vi "observacao_queued.vi"() -> ()   [LabVIEW 2012, in "Shared_160.lvlib"] (continued)
                w579 = u16 7 items=["Alarme", "Atencao", "Erro", "Ocupado", "TBD", "LCB", "Trapeira", "Paravento", "DomoRap", "DomoCW", "DomoCCW", "TBD", "Em movimento", "TBD"] ("NomeStatus")
                # "Aqui também caberia um Timeout?"
                # "Também poderia ser testado o bit \"Em movimento\".\nNeste caso o código do \"IF\" deve ser permutado."
                # "Aguarda abaixamento Paravento"
                n668 = call "Bit Status CUP.vi"("NomeStatus"=w579) -> ("StatBit"=w581:bool)
                n669 = case shown="True" w581 {
                  tunnel: [5 6] -> w580
                  frame False {
                    # "Ainda movendo...\nAGUARDAR"
                  }
                  frame True {
                    # "Paravento abaixado."
                  }
                }
              }
              frame 6 {
                w584 = u16 6 items=["Alarme", "Atencao", "Erro", "Ocupado", "TBD", "LCB", "Trapeira", "Paravento", "DomoRap", "DomoCW", "DomoCCW", "TBD", "Em movimento", "TBD"] ("NomeStatus")
                # "Verifica Trapeira"
                n670 = call "Bit Status CUP.vi"("NomeStatus"=w584) -> ("StatBit"=w585:bool)
                n671 = Not(x=w585) -> (.not. x?=w589:bool)
                n672 = And(x=w589, y="ChkOpenShutter") -> (x .and. y?=w587:bool)
                n673 = case shown="True" w587 {
                  tunnel: [0 w594] -> w590
                  tunnel: w586 -> [_ w595]
                  frame False {
                    # "Verificar Paravento"
                    # "Trapeira aberta\nou desabilitada"
                    n674 = call "TickTimeout.vi"() -> ("msTick"=w591:u32)  [unwired: 2 in, 2 out]
                    n675 = local write "TimeoutCUP"(w591) -> ()
                    n676 = global write "Global_Telescopio.vi" "T cup"(w591) -> ()
                    "Dome on Target" <- TRUE
                  }
                  frame True {
                    # "Abrir Trapeira"
                    n677 = case shown="False" w595 {
                      tunnel: [7 w600] -> w594
                      frame False {
                        w599 = u16 4 items=["ZERO", "AH", "DEC", "TUBO", "CUP"] ("Controlador")
                        # "Aguardar abertura Trap."
                        # "CLP Pronto"
                        n678 = call "Monta Comando.vi"("Comando"="ABRIR", "Dispositivo"="TRAPEIRA" ("Comando"), "Controlador"=w599) -> ()  [unwired: 4 in, 3 out]
                      }
                      frame True {
                        # "CLP Busy"
                        n679 = local read "TimeoutCUP"() -> (w602:u32)
                        n680 = call "TickTimeout.vi"("msInicial"=w602, "msTimeout"=u32 5000) -> ("Timeout"=w601:bool)  [unwired: 2 out]
                        n681 = case shown="True" w601 {
                          tunnel: [6 3] -> w600
                          frame False {
                          }
                          frame True {
                          }
                        }
                      }
                    }
                  }
                }
              }
              frame 7 {
                w606 = u16 6 items=["Alarme", "Atencao", "Erro", "Ocupado", "TBD", "LCB", "Trapeira", "Paravento", "DomoRap", "DomoCW", "DomoCCW", "TBD", "Em movimento", "TBD"] ("NomeStatus")
                # "Aqui também caberia um Timeout?"
                # "Aguarda abertura Trapeira"
                # "Também poderia ser testado o bit \"Em movimento\".\nNeste caso o código do \"IF\" deve ser permutado."
                n682 = call "Bit Status CUP.vi"("NomeStatus"=w606) -> ("StatBit"=w607:bool)
                n683 = case shown="True" w607 {
                  tunnel: [7 0] -> w608
                  frame False {
                    # "Ainda movendo...\nAGUARDAR"
                  }
                  frame True {
                    w611 = TRUE ("Dome on Target")
                    # "Trapeira aberta.\nFIM"
                    n684 = call "TickTimeout.vi"() -> ("msTick"=w610:u32)  [unwired: 2 in, 2 out]
                    n685 = local write "Dome on Target"(w611) -> ()
                    n686 = local write "RefreshShutterState"(w611) -> ()
                    n687 = local write "TimeoutCUP"(w610) -> ()
                    n688 = global write "Global_Telescopio.vi" "T cup"(w610) -> ()
                  }
                }
              }
            }
            n689 = case shown="True" w470 {
              tunnel: w459 -> [w490 _]
              tunnel: [w489 "POINT" ("Boolean Text.Text")] -> w458
              frame False {
                n690 = case shown="True" w490 {
                  tunnel: ["POINT" ("Boolean Text.Text") "STOP" ("Boolean Text.Text")] -> w489
                  frame False {
                  }
                  frame True {
                  }
                }
              }
              frame True {
                w493 = TRUE
                # "MUDANÇA:\n22/6/2011 \nHab. Guider"
                n691 = local read "ChkDomeEnable"() -> (w494:bool)
                n692 = global write "Global_Telescopio.vi" "Botão GO = STOP"(FALSE) -> ()
                n693 = local write "LED GUIDER"(w493) -> ()
                n694 = local write "GUIDER"(w493) -> ()
                n695 = local write "DOME"(w494) -> ()
              }
            }
            n696 = Tick Count (ms)() -> (millisecond timer value=w451:u32)
            n697 = Subtract(x=w451, y=w457) -> (x-y=w450:u32)
            n698 = Less?(x=w450, y=w452) -> (x < y?=w453:bool)
            n699 = control-ref of="BtTargetPoint"() -> (w487:refnum<vi>)
            n700 = case shown="True" w453 {
              tunnel: w452 -> [_ w488]
              frame False {
              }
              frame True {
                n701 = Wait Until Next ms Multiple(millisecond multiple=w488) -> ()  [unwired: 1 out]
              }
            }
            n702 = property class="Bool"(reference=w487, "Boolean Text.Text"=w458) -> ()  [unwired: 1 in, 2 out]
            n703 = call "PROTECAO.vi"("Estado In"=w463) -> ("Estado Out"=w462:i32)  [unwired: 2 in]
            n704 = local write "statCUP"(w462) -> ()
            "statCUP 2" <- "statCUP"
            "Erro Lim" <- 15 ("y")
            "Erro PROTEC" <- 10 ("y")
          }
          frame #4 {
            # "CHECA FINAL DO APONTAMENTO"
            # "ascensão reta = tempo sideral - ângulo horário (2)"
            n705 = local read "LedPointing"() -> (w909:bool)
            n706 = case shown="True" w909 {
              frame False {
                n707 = property on="DOME" class="Bool (strict)"("Disabled"=u8 0) -> ()  [unwired: 2 in, 2 out]
              }
              frame True {
                n708 = local read "statCUP"() -> (w914:i32)
                n709 = local read "statAH"() -> (w913:i32)
                n710 = local read "statDEC"() -> (w915:i32)
                n711 = Compound Arithmetic op=ADD(w914, w913, w915) -> (w916:i32)
                n712 = Greater Than 0?(x=w916) -> (x > 0?=w912:bool)
                n713 = case shown="False" w912 {
                  selector: w912 -> [w917 _]
                  frame False {
                    w920 = TRUE
                    n714 = local read "ChkPointPrecessed"() -> (w918:bool)
                    n715 = local read "StrPointObjName"() -> (w923:string)
                    n716 = local read "StrPointObjRA"() -> (w922:string)
                    n717 = local read "StrPointObjDEC"() -> (w921:string)
                    n718 = local write "LedPointing"(w917) -> ()
                    n719 = property on="LedPointing" class="Bool (strict)"("Visible"=w917) -> ()  [unwired: 2 in, 2 out]
                    n720 = case shown="True" w918 {
                      tunnel: ["2000.0" ("Saída") w925] -> w919
                      frame False {
                      }
                      frame True {
                        n721 = call "Calcula epoch.vi"() -> ("epoch"=w928:dbl)  [unwired: 2 in]
                        n722 = Number To Fractional String(number=w928, precision (6)=i16 1) -> (F-format string=w926:string)  [unwired: 2 in]
                        n723 = call "Comma_to_Point.vi"("Lat_A"=w926) -> ("Saída"=w925:string)
                      }
                    }
                    n724 = global write "Global_Telescopio.vi" "NAME OBJETO"(w923) -> ()
                    n725 = global write "Global_Telescopio.vi" "DEC AQUIS"(w921) -> ()
                    n726 = global write "Global_Telescopio.vi" "RA AQUIS"(w922) -> ()
                    n727 = local write "Processa Centragem"(w920) -> ()
                    n728 = property on="LedPointWorkArea" class="Bool (strict)"("Visible"=w920) -> ()  [unwired: 2 in, 2 out]
                    n729 = global write "Global_Telescopio.vi" "EPOCH AQUIS"(w919) -> ()
                  }
                  frame True {
                  }
                }
              }
            }
            n730 = local read "VARIABLE \nTRACKING"() -> (w910:bool)
            n731 = case shown="False" w910 {
              frame False {
              }
              frame True {
                n732 = local write "DEC"("DECTARGET") -> ()
                n733 = local write "RA"("AHTARGET") -> ()
              }
            }
          }
          frame #5 {
            # "PROCESSO OBJETO CENTRADO"
            n734 = case shown="True" "Processa Centragem" {
              frame False {
              }
              frame True {
                w937 = u16 3 items=["Alarme", "Atencao", "Erro", "Ocupado", "Protecao", "Embreagem", "Tracking", "Var. Track", "Rápido", "Ligeiro", "Médio", "Lento", "Em movimento", ""] ("NomeStatus")
                w938 = u16 3 items=["Alarme", "Atencao", "Erro", "Ocupado", "Protecao", "Embreagem", "Tracking", "Var. Track", "Rápido", "Ligeiro", "Médio", "Lento", "Em movimento", ""] ("NomeStatus")
                # "Roda case interno quando \nos controladores AH e DEC\nestiverem desocupados."
                n735 = call "Bit Status AH.vi"("NomeStatus"=w938) -> ("StatBit"=w936:bool)
                n736 = call "Bit Status DEC.vi"("NomeStatus"=w937) -> ("StatBit"=w935:bool)
                n737 = Or(x=w936, y=w935) -> (x .or. y?=w932:bool)
                n738 = case shown="False" w932 {
                  selector: w932 -> [w957 _]
                  tunnel: "INDEXER" ("Comando") -> [w959 _]
                  tunnel: "ZERAR" ("Comando") -> [w958 _]
                  frame False {
                    w945 = u16 1 items=["ZERO", "AH", "DEC", "TUBO", "CUP"] ("Controlador")
                    w946 = u16 2 items=["ZERO", "AH", "DEC", "TUBO", "CUP"] ("Controlador")
                    w939 = 0.0 ("AcumAG DEC")
                    # "PROCESSOPRECESSÃO"
                    # "PROCESSO ZERA POS_MOTOR"
                    # "Precessão"
                    n739 = local read "PM_RA"() -> (w951:string)
                    n740 = local read "Temp amb"() -> (w954:string)
                    n741 = local read "hum local"() -> (w952:string)
                    n742 = local read "MeanDEC"() -> (w955:string)
                    n743 = local read "pressão atm"() -> (w953:string)
                    n744 = local read "MeanRA"() -> (w956:string)
                    n745 = local read "PM_DEC"() -> (w950:string)
                    n746 = call "Monta Comando.vi"("Comando"=w958, "Dispositivo"=w959, "Controlador"=w945) -> ()  [unwired: 4 in, 3 out]
                    n747 = call "Monta Comando.vi"("Comando"=w958, "Dispositivo"=w959, "Controlador"=w946) -> ()  [unwired: 4 in, 3 out]
                    n748 = call "PrecessFortran.vi"("Asc reta"=w956, "Var RA"=w951, "Declinação"=w955, "Temperatura (Kelvin)"=w954, "Pressao atmosferica (mB)"=w953, "Humidade relativa (0 a 1)"=w952, "Var DEC"=w950) -> ("Observed RA (radians)"=w949:dbl, "Observed Dec (radians)"=w948:dbl)  [unwired: 2 in, 5 out]
                    n749 = local write "Processa Centragem"(w957) -> ()
                    n750 = global write "Global_Telescopio.vi" "LatchPrecRA"(w949) -> ()
                    n751 = global write "Global_Telescopio.vi" "LatchPrecDEC"(w948) -> ()
                    n752 = global read "Global_Telescopio.vi" "Sideral Time"() -> (w942:dbl)
                    n753 = global read "Global_Telescopio.vi" "PosDEC"() -> (w944:dbl)
                    n754 = global read "Global_Telescopio.vi" "PosAH"() -> (w943:dbl)
                    n755 = Subtract(x=w942, y=w943) -> (x-y=w941:dbl)
                    n756 = local write "LatchDeslocDEC"(w944) -> ()
                    n757 = local write "LatchDeslocRA"(w941) -> ()
                    n758 = global write "Global_Telescopio.vi" "AcumPrecDEC"(w939) -> ()
                    n759 = global write "Global_Telescopio.vi" "LatchAG RA"(w939) -> ()
                    n760 = global write "Global_Telescopio.vi" "AcumAG DEC"(w939) -> ()
                    n761 = global write "Global_Telescopio.vi" "AcumPrecRA"(w939) -> ()
                    n762 = global write "Global_Telescopio.vi" "LatchAG DEC"(w939) -> ()
                    n763 = global write "Global_Telescopio.vi" "AcumAG RA"(w939) -> ()
                    n764 = global write "Global_Telescopio.vi" "ObjCentrado"(TRUE) -> ()
                    n765 = property on="Calagem" class="Bool"("Disabled"=u8 0) -> ()  [unwired: 2 in, 2 out]
                  }
                  frame True {
                  }
                }
              }
            }
          }
          frame #6 {
            w963 = u16 2 items=["Alarme", "Atencao", "Erro", "Ocupado", "TBD", "LCB", "Trapeira", "Paravento", "DomoRap", "DomoCW", "DomoCCW", "TBD", "Em movimento", "TBD"] ("NomeStatus")
            w964 = u16 3 items=["Alarme", "Atencao", "Erro", "Ocupado", "TBD", "LCB", "Trapeira", "Paravento", "DomoRap", "DomoCW", "DomoCCW", "TBD", "Em movimento", "TBD"] ("NomeStatus")
            w968 = u16 3 items=["Alarme", "Atencao", "Erro", "Ocupado", "Protecao", "Embreagem", "Tracking", "Var. Track", "Rápido", "Ligeiro", "Médio", "Lento", "Em movimento", ""] ("NomeStatus")
            w969 = u16 3 items=["Alarme", "Atencao", "Erro", "Ocupado", "Protecao", "Embreagem", "Tracking", "Var. Track", "Rápido", "Ligeiro", "Médio", "Lento", "Em movimento", ""] ("NomeStatus")
            w977 = "ERROS" ("Comando")
            w980 = u16 2 items=["Alarme", "Atencao", "Erro", "Ocupado", "Protecao", "Embreagem", "Tracking", "Var. Track", "Rápido", "Ligeiro", "Médio", "Lento", "Em movimento", ""] ("NomeStatus")
            w981 = u16 2 items=["Alarme", "Atencao", "Erro", "Ocupado", "Protecao", "Embreagem", "Tracking", "Var. Track", "Rápido", "Ligeiro", "Médio", "Lento", "Em movimento", ""] ("NomeStatus")
            w978 = "PROG" ("Comando")
            # "LOGTCS ERROS"
            n766 = call "Bit Status AH.vi"("NomeStatus"=w981) -> ("StatBit"=w971:bool)
            n767 = call "Bit Status AH.vi"("NomeStatus"=w969) -> ("StatBit"=w967:bool)
            n768 = call "Bit Status DEC.vi"("NomeStatus"=w980) -> ("StatBit"=w970:bool)
            n769 = call "Bit Status DEC.vi"("NomeStatus"=w968) -> ("StatBit"=w966:bool)
            n770 = call "Bit Status CUP.vi"("NomeStatus"=w963) -> ("StatBit"=w979:bool)
            n771 = call "Bit Status CUP.vi"("NomeStatus"=w964) -> ("StatBit"=w976:bool)
            n772 = Not(x=w976) -> (.not. x?=w975:bool)
            n773 = Not(x=w967) -> (.not. x?=w973:bool)
            n774 = Not(x=w966) -> (.not. x?=w974:bool)
            n775 = And(x=w979, y=w975) -> (x .and. y?=w962:bool)
            n776 = And(x=w971, y=w973) -> (x .and. y?=w972:bool)
            n777 = And(x=w970, y=w974) -> (x .and. y?=w965:bool)
            n778 = And(x=FALSE, y=w962) -> (x .and. y?=w961:bool)
            n779 = case shown="True" w965 {
              selector: w965 -> [_ w990]
              tunnel: w978 -> [_ w991]
              tunnel: w977 -> [_ w987]
              frame False {
              }
              frame True {
                w988 = u16 2 items=["ZERO", "AH", "DEC", "TUBO", "CUP"] ("Controlador")
                n780 = call "Monta Comando.vi"("Comando"=w987, "Dispositivo"=w991, "Controlador"=w988) -> ("Resposta"=w989:string)  [unwired: 4 in, 2 out]
                n781 = call "Envia LOG.vi"("Error message"=w989, "Controlador"=w988, "Log de erro"=w990) -> ()  [unwired: 5 in, 2 out]
              }
            }
            n782 = case shown="True" w961 {
              selector: w961 -> [_ w985]
              tunnel: w978 -> [_ w986]
              tunnel: w977 -> [_ w982]
              frame False {
              }
              frame True {
                w983 = u16 4 items=["ZERO", "AH", "DEC", "TUBO", "CUP"] ("Controlador")
                n783 = call "Monta Comando.vi"("Comando"=w982, "Dispositivo"=w986, "Controlador"=w983) -> ("Resposta"=w984:string)  [unwired: 4 in, 2 out]
                n784 = call "Envia LOG.vi"("Error message"=w984, "Controlador"=w983, "Log de erro"=w985) -> ()  [unwired: 5 in, 2 out]
              }
            }
            n785 = case shown="True" w972 {
              selector: w972 -> [_ w995]
              tunnel: w978 -> [_ w996]
              tunnel: w977 -> [_ w992]
              frame False {
              }
              frame True {
                w993 = u16 1 items=["ZERO", "AH", "DEC", "TUBO", "CUP"] ("Controlador")
                n786 = call "Monta Comando.vi"("Comando"=w992, "Dispositivo"=w996, "Controlador"=w993) -> ("Resposta"=w994:string)  [unwired: 4 in, 2 out]
                n787 = call "Envia LOG.vi"("Error message"=w994, "Controlador"=w993, "Log de erro"=w995) -> ()  [unwired: 5 in, 2 out]
              }
            }
          }
          frame #7 {
            # "MASSA DE AR"
            # "z'"
            # "z * (1 - 0,0012* (z* z -1) )"
            # "(z* z -1)"
            # "z"
            # "O Hour Angle é calculado com essa equação (AH = TS - RA), \nsendo TS o tempo sideral que você fica calculando o tempo todo e RA a \ncoordenada que vem do quadro TARGET da aba POINTING."
            # "Coslat"
            # "Sinlat"
            # "MASSA DE AR\n# define LAT -22,534444444444 / / Lat itude do telescópio\n# define SINLAT -0,383238771 / / Seno da Lat itude\n# define COSLAT 0,923649308 / / Cosseno da Lat itude\ndouble airmass (double ah, double delta) / / ângulos dos eixos AH e DEC em radianos\n{ double z;\nz = 1./ (SINLAT* sin(delta) + COSLAT* cos(delta) * cos(ah) ) ;\nz = z * (1 - 0,0012* (z* z -1) ) ;\nif (z > = 10) z = 9.999;\nif (z < 0) z = 0;\nreturn (z) ;\n}"
            n788 = global read "Global_Telescopio.vi" "AH_now"() -> (w997:dbl)
            n789 = global read "Global_Telescopio.vi" "delta_now"() -> (w998:dbl)
            n790 = Cosine(x=w998) -> (cos(x)=w1018:dbl)
            n791 = Sine(x=w998) -> (sin(x)=w1020:dbl)
            n792 = Cosine(x=w997) -> (cos(x)=w1016:dbl)
            n793 = Multiply(x=0.923649308 ("Delta=DEC"), y=w1018) -> (x*y=w1017:dbl)
            n794 = Multiply(x=-0.383238771 ("Delta=DEC"), y=w1020) -> (x*y=w1015:dbl)
            n795 = Multiply(x=w1017, y=w1016) -> (x*y=w1014:dbl)
            n796 = Add(x=w1015, y=w1014) -> (x+y=w1013:dbl)
            n797 = Reciprocal(x=w1013) -> (1/x=w1005:dbl)
            n798 = Subtract(x=w1005, y=1.0) -> (x-y=w1011:dbl)
            n799 = Multiply(x=w1005, y=w1011) -> (x*y=w1010:dbl)
            n800 = Multiply(x=w1010, y=0.0012) -> (x*y=w1007:dbl)
            n801 = Subtract(x=1.0 ("y"), y=w1007) -> (x-y=w1006:dbl)
            n802 = Multiply(x=w1005, y=w1006) -> (x*y=w1002:dbl)
            n803 = Greater Or Equal?(x=w1002, y=10.0) -> (x >= y?=w1003:bool)
            n804 = case shown="True" w1003 {
              tunnel: [w1024 9.999999 ("y")] -> w1000
              tunnel: w1002 -> [w1024 _]
              frame False {
              }
              frame True {
              }
            }
            n805 = Less Than 0?(x=w1000) -> (x < 0?=w1001:bool)
            n806 = case shown="True" w1001 {
              tunnel: [w1022 0.0 ("y")] -> w999
              tunnel: w1000 -> [w1022 _]
              frame False {
              }
              frame True {
              }
            }
            "Air Mass" <- w999
            n807 = global write "Global_Telescopio.vi" "Air Mass"(w999) -> ()
          }
          frame #8 {
          }
          frame #9 {
            # "CONDIÇÕES ATMOSFÉRICAS"
            # "Se mudou a Chave\ngera um Pulso"
            # "A cada n Segundos\nEssa rotina gera 1\npulso!"
            # "Seg"
            # "Janela Das Condições Atmosféricas"
            n808 = local read "Int/Ext"() -> (w1028:bool)
            n809 = global read "Global_Telescopio.vi" "Default Met"() -> (w1026:bool)
            n810 = call "timepulse.vi"("de quantos segundos"=i16 10) -> ("PULSO"=w1032:bool)  [unwired: 2 in]
            n811 = call "Pulso_se_Mudou.vi"("Entrada"=w1028) -> ("Saída"=w1029:bool)
            n812 = local write "Default Met"(w1026) -> ()
            n813 = Or(x=w1029, y=w1032) -> (x .or. y?=w1030:bool)
            n814 = case shown="True" w1030 {
              tunnel: [_ TRUE ("Int/Ext")] -> w1027
              frame False {
              }
              frame True {
                n815 = stacked-sequence {
                  frame #0 {
                    # "O botão INT/ EXT (cf. figura 3) seleciona se os most radores TEMPERATURE, HUMIDITY\ne DEW POINT são atualizados com os valores internos ou externos desse regist ro.\nA barra gráfica CLOUSURE LIMITS deve ser deslocada em função da proximidade\n(dada por um valor percentural de zero a 100%) dos valores lidos do arquivo de dados\natmosféricos com os valores- limite das grandezas listadas nesse quadro. Para\nPRESSURE e WIND SPEED, considerar os valores- limite desse quadro como o final de\numa escala de 0 a 100%, cujo valor inicial (0%) corresponde ao valor zero dessas\ngrandezas. Para as grandezas DEWPOINT, interna e externa, considerar os valores\nlimites listados no quadro como final da escala (100%) e cada décimo de ºC acima\ndos valores- limite como 1% da escala."
                    # "A simulação da janela ENVIRONMENT STATUS será feita com os dados de um arquivo\ngerado pela estação meteorológica contendo os regist ros de 24 horas de monitoria,\nsendo cada regist ro efetuado em intervalos de 10 minutos. A simulação deve procurar\nnesse arquivo (anexo, LNA-TCSPD-MP-00012-01-100.txt ) o regist ro correspondente à\nhora local do PC, ler esse regist ro e ret irar as informações de cada most rador para\natualizar essa janela."
                  }
                  frame #1 {
                    w1044 = "\t"
                    (unwired) "1:04" ("Hora a ser Procurada")
                    # "Lê arquivo, da Est. Meteor."
                    # "MUDANÇA FUTURA:\nSe possível, mostrar os valores de Pressão atm,\nTemp. amb. e umidade rel.\nda estação do tubo em lugar\ndos valores internos."
                    # "O Fortran usa valores\nde umidade entre 0 e 1."
                    # "MUDANÇA 08/04/2011:\nCriada a variável AtmosferaStr para guardar dados\nmeteorológicos para Erros de Apontamento"
                    # "Celsius -->Kelvin\nO Fortran usa Kelvin"
                    # "bar"
                    # "Formato"
                    n816 = case shown="False" "Default Met" {
                      tunnel: ["OFF" "ON"] -> w1042
                      frame False {
                      }
                      frame True {
                      }
                    }
                    n817 = case shown="True" "Int/Ext" {
                      tunnel: [27 ("index") 2 ("index")] -> w1076
                      tunnel: [28 ("index") 5 ("index")] -> w1075
                      tunnel: [29 ("index") 6 ("index")] -> w1074
                      frame False {
                        # "Interno"
                      }
                      frame True {
                        # "Externo"
                      }
                    }
                    n818 = property on="Default" class="Str"("Visible"="Default Met") -> ()  [unwired: 2 in, 2 out]
                    n819 = global write "Global_Telescopio.vi" "WS_DEFAULT"(w1042) -> ()
                    n820 = case shown="False" "Default Met" {
                      tunnel: [w1103 string[] ["24/05/18", "13:00", "19.1", "19.1", "19.1", "61", "11.4", "2.2", "NNW", "0.67", "4.5", "NNW", "19.1", "18.8", "18.8", "24.1", "761.5", "0.00", "0.0", "705", "5.05", "710", "5.9", "0.21", "5.9", "0.000", "0.003", "17.6", "53", "7.9", "16.7", "20.6", "16.7", "40", "50", "0.43", "0", "113", "1", "99.1", "5", "\r\n", "", "", "", "", ""] ("Array")] -> w1099
                      frame False {
                        n821 = call "Procura_no_Arquivo.vi"() -> ("Erro de Leitura=True"=w1102:bool, "Array"=w1103:string[])  [unwired: 4 in]
                        n822 = local write "Default Met"(w1102) -> ()
                      }
                      frame True {
                      }
                    }
                    n823 = Index Array(array=w1099, index #1=w1076, index #2=w1075, index #3=w1074, index #4=7 ("index"), index #5=8 ("index"), index #6=12 ("index"), index #7=16 ("index"), index #8=2 ("index"), index #9=5 ("index"), index #10=27 ("index"), index #11=28 ("index"), index #12=36 ("index")) -> (element #1=w1085:string, element #2=w1098:string, element #3=w1095:string, element #4=w1091:string, element #5=w1045:string, element #6=w1090:string, element #7=w1086:string, element #8=w1059:string, element #9=w1058:string, element #10=w1055:string, element #11=w1054:string, element #12=w1036:string)
                    "Wind Dir" <- w1045
                    n824 = Decimal String To Number(string=w1036) -> (number=→"LEAF":i32)  [unwired: 2 in, 1 out]
                    n825 = call "point_to_comma.vi"("Lat_A"=w1085) -> ("Saída"=w1081:string)
                    n826 = call "point_to_comma.vi"("Lat_A"=w1098) -> ("Saída"=w1082:string)
                    n827 = call "point_to_comma.vi"("Lat_A"=w1095) -> ("Saída"=w1048:string)
                    n828 = call "point_to_comma.vi"("Lat_A"=w1091) -> ("Saída"=w1046:string)
                    n829 = call "point_to_comma.vi"("Lat_A"=w1090) -> ("Saída"=w1047:string)
                    n830 = call "point_to_comma.vi"("Lat_A"=w1086) -> ("Saída"=w1051:string)
                    "pressão atm" <- w1051
                    n831 = call "point_to_comma.vi"("Lat_A"=w1059) -> ("Saída"=w1053:string)
                    n832 = call "point_to_comma.vi"("Lat_A"=w1058) -> ("Saída"=w1052:string)
                    n833 = call "point_to_comma.vi"("Lat_A"=w1055) -> ("Saída"=w1050:string)
                    n834 = call "point_to_comma.vi"("Lat_A"=w1054) -> ("Saída"=w1049:string)
                    n835 = Concatenate Strings(w1053, w1044, w1052, w1044, w1051, w1044, w1050, w1044, w1049, w1044, w1048, w1044, w1046, w1044, w1045, w1044) -> (→"AtmosferaStr":string)
                    n836 = Fract/Exp String To Number(string=w1081, default (0 dbl)=1.0 ("default (0 DBL)")) -> (number=w1041:dbl)  [unwired: 2 in, 1 out]
                    "Temperature" <- w1041
                    n837 = Fract/Exp String To Number(string=w1082, default (0 dbl)=1.0 ("default (0 DBL)")) -> (number=w1040:dbl)  [unwired: 2 in, 1 out]
                    "Humidity" <- w1040
                    n838 = Fract/Exp String To Number(string=w1048, default (0 dbl)=1.0 ("default (0 DBL)")) -> (number=→"Dew Point":dbl)  [unwired: 2 in, 1 out]
                    n839 = Fract/Exp String To Number(string=w1046, default (0 dbl)=1.0 ("default (0 DBL)")) -> (number=→"Wind Speed":dbl)  [unwired: 2 in, 1 out]
                    n840 = Fract/Exp String To Number(string=w1047, default (0 dbl)=1.0 ("default (0 DBL)")) -> (number=→"Wind Chill":dbl)  [unwired: 2 in, 1 out]
                    n841 = Fract/Exp String To Number(string=w1051, default (0 dbl)=1.0 ("default (0 DBL)")) -> (number=w1039:dbl)  [unwired: 2 in, 1 out]
                    "Pressure" <- w1039
                    n842 = Fract/Exp String To Number(string=w1053, default (0 dbl)=1.0 ("default (0 DBL)")) -> (number=w1062:dbl)  [unwired: 2 in, 1 out]
                    n843 = Fract/Exp String To Number(string=w1052, default (0 dbl)=1.0 ("default (0 DBL)")) -> (number=w1061:dbl)  [unwired: 2 in, 1 out]
                    n844 = Add(x=w1062, y=273.5 ("default (0 DBL)")) -> (x+y=w1079:dbl)
                    n845 = Divide(x=w1061, y=100.0 ("default (0 DBL)")) -> (x/y=w1064:dbl)
                    n846 = global write "Global_Telescopio.vi" "BAR"(w1039) -> ()
                    n847 = global write "Global_Telescopio.vi" "HUM"(w1040) -> ()
                    n848 = global write "Global_Telescopio.vi" "TEMP"(w1041) -> ()
                    n849 = Number To Fractional String(number=w1079, precision (6)=i16 1) -> (F-format string=→"Temp amb":string)  [unwired: 2 in]
                    n850 = Number To Fractional String(number=w1064, precision (6)=i16 2) -> (F-format string=→"hum local":string)  [unwired: 2 in]
                  }
                  frame #2 {
                    # "Em relação as suas perguntas:\n- Temperaturas (Temperature, Dew Point e Wind Chill): mínimo/máximo: -20 a +50 graus\n- Humidity:  0 a 100%\n- Pressão atmosférica: de 300 a 1200 mBar\n- Velocidade do vento: 0 a 300 Km/h\n\nNotar que a chave INT/EXT na parte superior do quadro \nesquerdo seleciona se são mostrados os valores internos ou externos de Temperatura, Umidade e Dew Point."
                    # "Pressure Max"
                    # "Wind chill Point Max"
                    # "Temp Point Max"
                    # "Dew Point Max"
                    # "Humidity Max"
                    # "Speed Max"
                    # "Steady Wind           >  70 Km/h\nRelative Humidity    >  97 %\nInternal Dewpoint  <  0.5  C\nExternal Dewpoint <  1.0  C"
                    n851 = Divide(x=100.0, y=300.0 ("x")) -> (x/y=w1142:dbl)
                    n852 = local read "Wind Speed"() -> (w1141:dbl)
                    n853 = Divide(x=100.0, y=100.0 ("x")) -> (x/y=w1136:dbl)
                    n854 = local read "Humidity"() -> (w1135:dbl)
                    n855 = local read "Dew Point"() -> (w1131:dbl)
                    n856 = Divide(x=100.0, y=50.0 ("x")) -> (x/y=w1128:dbl)
                    n857 = Divide(x=100.0, y=1200.0 ("x")) -> (x/y=w1122:dbl)
                    n858 = Divide(x=100.0, y=50.0 ("x")) -> (x/y=w1134:dbl)
                    n859 = Divide(x=100.0, y=50.0 ("x")) -> (x/y=w1127:dbl)
                    n860 = Multiply(x=w1141, y=w1142) -> (x*y=w1118:dbl)
                    n861 = local read "Temperature"() -> (w1119:dbl)
                    n862 = local read "Wind Chill"() -> (w1120:dbl)
                    n863 = local read "Pressure"() -> (w1121:dbl)
                    n864 = Multiply(x=w1135, y=w1136) -> (x*y=w1117:dbl)
                    n865 = Multiply(x=w1119, y=w1128) -> (x*y=w1115:dbl)
                    n866 = Multiply(x=w1121, y=w1122) -> (x*y=w1113:dbl)
                    n867 = Multiply(x=w1131, y=w1134) -> (x*y=w1116:dbl)
                    n868 = Multiply(x=w1120, y=w1127) -> (x*y=w1114:dbl)
                    n869 = Build Array(w1118, w1117, w1116, w1115, w1114, w1113) -> (w1112:dbl[])
                    n870 = Array Max & Min(array=w1112) -> (max value=w1111:dbl)  [unwired: 3 out]
                    n871 = local write "SlideEnviromental"(w1111) -> ()
                  }
                  frame #3 {
                    # "Determinadas as proximidades de cada grandeza em valores percentuais, selecionar o\nvalor da mais elevada para ser most rado na barra gráfica. A cor dessa barra gráfica\ndeve mudar em função do valor most rado. Enquanto est iver abaixo de 90%, ela deve\nser verde, ent re 90 e 95% amarela e acima de 95% vermelha. O led ao lado desse\nbarra deve ficar ligado e ter a mesma cor da barra gráfica, mas quando esta\nult rapassar 90%, ou seja quando for amarela ou vermelha, o led deve piscar."
                    n872 = local read "SlideEnviromental"() -> (w1143:dbl)
                    n873 = In Range and Coerce(upper limit=95.0 ("lower limit"), x=w1143, lower limit=90.0 ("upper limit")) -> (In Range?=w1148:bool)  [unwired: 1 out]
                    n874 = Less?(x=w1143, y=90.0) -> (x < y?=w1150:bool)
                    n875 = Greater?(x=w1143, y=95.0 ("lower limit")) -> (0:w1147:bool)
                    n876 = case shown="True" w1148 {
                      frame False {
                      }
                      frame True {
                        n877 = stacked-sequence {
                          frame #0 {
                            n878 = property on="SlideEnviromental" class="Slide (strict)"("Fill Color"=u32 16772882) -> ()  [unwired: 2 in, 2 out]
                            n879 = local write "Boolean 11"(TRUE ("Boolean 11")) -> ()
                            n880 = property on="Boolean 11" class="Bool (strict)"("Blinking"=FALSE) -> ()  [unwired: 2 in, 2 out]
                          }
                          frame #1 {
                            # "Cor do Led"
                            # "lig"
                            # "des"
                            n881 = Bundle(u32 7171459, u32 46096) -> (w1170:cluster{u32, u32})  [unwired: 1 in]
                            n882 = Bundle(u32 16772882, u32 46096) -> (w1169:cluster{u32, u32})  [unwired: 1 in]
                            n883 = Build Array(w1170, w1169) -> (w1168:cluster{u32, u32}[])
                            n884 = property on="Boolean 11" class="Bool (strict)"("Colors [4]"=w1168) -> ()  [unwired: 2 in, 2 out]
                          }
                        }
                      }
                    }
                    n885 = case shown="True" w1150 {
                      frame False {
                      }
                      frame True {
                        n886 = stacked-sequence {
                          frame #0 {
                            n887 = property on="SlideEnviromental" class="Slide (strict)"("Fill Color"=u32 6618880) -> ()  [unwired: 2 in, 2 out]
                            n888 = local write "Boolean 11"(TRUE ("Boolean 11")) -> ()
                            n889 = property on="Boolean 11" class="Bool (strict)"("Blinking"=FALSE) -> ()  [unwired: 2 in, 2 out]
                          }
                          frame #1 {
                            # "Cor do Led"
                            # "lig"
                            # "des"
                            n890 = Bundle(u32 7171459, u32 46096) -> (w1174:cluster{u32, u32})  [unwired: 1 in]
                            n891 = Bundle(u32 6618880, u32 46096) -> (w1175:cluster{u32, u32})  [unwired: 1 in]
                            n892 = Build Array(w1174, w1175) -> (w1176:cluster{u32, u32}[])
                            n893 = property on="Boolean 11" class="Bool (strict)"("Colors [4]"=w1176) -> ()  [unwired: 2 in, 2 out]
                          }
                        }
                      }
                    }
                    n894 = case shown="True" w1147 {
                      frame False {
                      }
                      frame True {
                        n895 = stacked-sequence {
                          frame #0 {
                            n896 = local write "Boolean 11"(TRUE ("Boolean 11")) -> ()
                            n897 = property on="SlideEnviromental" class="Slide (strict)"("Fill Color"=u32 16715776) -> ()  [unwired: 2 in, 2 out]
                            n898 = property on="Boolean 11" class="Bool (strict)"("Blinking"=TRUE) -> ()  [unwired: 2 in, 2 out]
                          }
                          frame #1 {
                            # "Cor do Led"
                            # "lig"
                            # "des"
                            n899 = Bundle(u32 7171459, u32 46096) -> (w1154:cluster{u32, u32})  [unwired: 1 in]
                            n900 = Bundle(u32 16715776, u32 46096) -> (w1155:cluster{u32, u32})  [unwired: 1 in]
                            n901 = Build Array(w1154, w1155) -> (w1156:cluster{u32, u32}[])
                            n902 = property on="Boolean 11" class="Bool (strict)"("Colors [4]"=w1156) -> ()  [unwired: 2 in, 2 out]
                          }
                        }
                      }
                    }
                  }
                }
              }
            }
            n903 = flat-sequence {
              tunnel: w1027 -> [_]
              frame #0 {
                n904 = local read "LEAF"() -> (w1033:i32)
                n905 = call "Testa_Leaf.vi"("LEAF"=w1033) -> ()  [unwired: 11 in]
              }
            }
          }
          frame #10 {
            w1191 = u16 3 items=["Alarme", "Atencao", "Erro", "Ocupado", "Protecao", "Embreagem", "Tracking", "Var. Track", "Rápido", "Ligeiro", "Médio", "Lento", "Em movimento", ""] ("NomeStatus")
            w1192 = u16 3 items=["Alarme", "Atencao", "Erro", "Ocupado", "Protecao", "Embreagem", "Tracking", "Var. Track", "Rápido", "Ligeiro", "Médio", "Lento", "Em movimento", ""] ("NomeStatus")
            # "PROCESSO AUTO GUIDER"
            n906 = local read "MOUNT"() -> (w1188:bool)
            n907 = local read "LedPointing"() -> (w1186:bool)
            n908 = global read "Global_Telescopio.vi" "Correção Guider"() -> (w1182:bool)
            n909 = local read "MOVING"() -> (w1185:bool)
            n910 = call "Bit Status AH.vi"("NomeStatus"=w1192) -> ("StatBit"=w1189:bool)
            n911 = call "Bit Status DEC.vi"("NomeStatus"=w1191) -> ("StatBit"=w1190:bool)
            n912 = Not(x=w1185) -> (.not. x?=w1184:bool)
            n913 = Not(x=w1186) -> (.not. x?=w1183:bool)
            n914 = Not Or(1:w1190, 2:w1189) -> (0:w1187:bool)
            n915 = Compound Arithmetic op=AND(w1182, w1183, w1184, "GUIDER", w1188, w1187) -> (w1193:bool)
            n916 = case shown="True" w1193 {
              frame False {
                # "Reseta Flag da comunicação do Guider"
                n917 = global write "Global_Telescopio.vi" "Correção Guider"(FALSE ("Correção Guider")) -> ()
              }
              frame True {
                # "MUDANÇA:\n(25/08/2010)"
                # "É necessário testar se as\nstrings são igual a espaço\nem virtude de um BUG,\nno Soft do Auto guider!"
                n918 = global read "Global_Telescopio.vi" "guide_dir_ns"() -> (w1200:string)
                n919 = global read "Global_Telescopio.vi" "guide_dir_we"() -> (w1201:string)
                n920 = case shown="\"W\"" w1201 {
                  tunnel: [0.0 ("PreciseOffsetDEC 2") 1.0 ("PreciseOffsetDEC 2") -1.0 ("PreciseOffsetDEC 2")] -> w1198
                  frame " ", Default {
                  }
                  frame "W" {
                  }
                  frame "E" {
                  }
                }
                n921 = case shown="\"N\"" w1200 {
                  tunnel: [0.0 ("PreciseOffsetDEC 2") 1.0 ("PreciseOffsetDEC 2") -1.0 ("PreciseOffsetDEC 2")] -> w1197
                  frame " ", Default {
                  }
                  frame "N" {
                  }
                  frame "S" {
                  }
                }
                n922 = Equal To 0?(x=w1198) -> (x = 0?=w1195:bool)
                n923 = Equal To 0?(x=w1197) -> (x = 0?=w1196:bool)
                n924 = And(x=w1195, y=w1196) -> (x .and. y?=w1199:bool)
                n925 = case shown="False" w1199 {
                  tunnel: w1198 -> [w1206 _]
                  tunnel: w1197 -> [w1205 _]
                  frame False {
                    # "Comandos do Auto guider contendo direção"
                    n926 = global read "Global_Telescopio.vi" "esc_placa"() -> (w1204:string)
                    n927 = Fract/Exp String To Number(use system decimal point (T)=FALSE, string=w1204) -> (number=w1203:dbl)  [unwired: 2 in, 1 out]
                    n928 = stacked-sequence {
                      tunnel: w1206 -> [w1212 _ _]
                      tunnel: w1205 -> [_ w1232 _]
                      tunnel: w1203 -> [w1209 w1229 _]
                      frame #0 {
                        n929 = local read "AtualDEC"() -> (w1217:dbl)
                        n930 = global read "Global_Telescopio.vi" "CorrecaoMin"() -> (w1207:dbl)
                        n931 = global read "Global_Telescopio.vi" "guide_asc"() -> (w1211:dbl)
                        n932 = Cosine(x=w1217) -> (cos(x)=w1216:dbl)
                        n933 = Multiply(x=w1211, y=w1209) -> (x*y=w1210:dbl)
                        n934 = Absolute Value(x=w1216) -> (abs(x)=w1215:dbl)
                        n935 = Divide(x=w1210, y=w1215) -> (x/y=w1213:dbl)
                        n936 = Multiply(x=w1212, y=w1213) -> (x*y=w1208:dbl)
                        n937 = Greater?(x=w1213, y=w1207) -> (0:w1214:bool)
                        n938 = case shown="True" w1214 {
                          tunnel: w1208 -> [_ w1219]
                          frame False {
                          }
                          frame True {
                            w1223 = u16 1 items=["ZERO", "AH", "DEC", "TUBO", "CUP"] ("Controlador")
                            # "PROCESSO MOVE TELESCÓPIO"
                            n939 = local read "Offset RA"() -> (w1220:dbl)
                            n940 = Add(x=w1219, y=w1220) -> (x+y=w1221:dbl)
                            n941 = property on="Calagem" class="Bool"("Disabled"=u8 2) -> ()  [unwired: 2 in, 2 out]
                            n942 = call "Conversao Ms to Hora texto.vi"("TRUE=HORA\nFALSE=GRAU"=TRUE ("TRUE=HORA\nFALSE=GRAU"), "PrecDEC"=w1219) -> ("Hora/Graus Texto Decimal"=w1226:string)
                            n943 = local write "Offset RA"(w1221) -> ()
                            n944 = call "Monta Comando.vi"("Set Point"=w1226, "Comando"="MOVER_REL", "Dispositivo"="EIXO" ("Comando"), "Controlador"=w1223) -> ()  [unwired: 3 in, 3 out]
                          }
                        }
                      }
                      frame #1 {
                        n945 = global read "Global_Telescopio.vi" "guide_dec"() -> (w1231:dbl)
                        n946 = Multiply(x=w1231, y=w1229) -> (x*y=w1230:dbl)
                        n947 = global read "Global_Telescopio.vi" "CorrecaoMin"() -> (w1227:dbl)
                        n948 = Greater?(x=w1230, y=w1227) -> (0:w1233:bool)
                        n949 = Multiply(x=w1232, y=w1230) -> (x*y=w1228:dbl)
                        n950 = case shown="True" w1233 {
                          tunnel: w1228 -> [_ w1235]
                          frame False {
                          }
                          frame True {
                            w1239 = u16 2 items=["ZERO", "AH", "DEC", "TUBO", "CUP"] ("Controlador")
                            # "PROCESSO MOVE TELESCÓPIO"
                            n951 = local read "Offset DEC"() -> (w1236:dbl)
                            n952 = Add(x=w1235, y=w1236) -> (x+y=w1237:dbl)
                            n953 = property on="Calagem" class="Bool"("Disabled"=u8 2) -> ()  [unwired: 2 in, 2 out]
                            n954 = call "Conversao Ms to Hora texto.vi"("TRUE=HORA\nFALSE=GRAU"=FALSE ("TRUE=HORA\nFALSE=GRAU"), "PrecDEC"=w1235) -> ("Hora/Graus Texto Decimal"=w1242:string)
                            n955 = local write "Offset DEC"(w1237) -> ()
                            n956 = call "Monta Comando.vi"("Set Point"=w1242, "Comando"="MOVER_REL", "Dispositivo"="EIXO" ("Comando"), "Controlador"=w1239) -> ()  [unwired: 3 in, 3 out]
                          }
                        }
                      }
                      frame #2 {
                        # "Reseta Flag da comunicação do Guider"
                        n957 = global write "Global_Telescopio.vi" "Correção Guider"(FALSE ("Correção Guider")) -> ()
                      }
                    }
                  }
                  frame True {
                  }
                }
              }
            }
            "LED GUIDER" <- "GUIDER"
          }
          frame #11 {
            w1259 = u16 12 items=["Alarme", "Atencao", "Erro", "Ocupado", "Protecao", "Embreagem", "Tracking", "Var. Track", "Rápido", "Ligeiro", "Médio", "Lento", "Em movimento", ""] ("NomeStatus")
            w1258 = u16 12 items=["Alarme", "Atencao", "Erro", "Ocupado", "Protecao", "Embreagem", "Tracking", "Var. Track", "Rápido", "Ligeiro", "Médio", "Lento", "Em movimento", ""] ("NomeStatus")
            # "Aqui era a Global\nLIMITE"
            # "Este teste deve ser executado antes do Frame de enviar\ncomando do sistema de aquisição, em virtude de teste do \nmovimento."
            # "Quando o Movimento Parar\nreseta a Variável/Flag para enviar \no CR ao sitema de Aquisição"
            n958 = global read "Global_Telescopio.vi" "AQ Offset Mov"() -> (w1255:bool)
            n959 = call "Bit Status AH.vi"("NomeStatus"=w1258) -> ("StatBit"=w1261:bool)
            n960 = call "Bit Status DEC.vi"("NomeStatus"=w1259) -> ("StatBit"=w1260:bool)
            n961 = local read "Proteção"() -> (w1251:bool)
            n962 = Not Or(1:w1260, 2:w1261) -> (0:w1256:bool)
            n963 = case shown="True" w1251 {
              selector: w1251 -> [w1262 w1263]
              frame False {
                n964 = local write "LIMITE"(w1262) -> ()
                n965 = property on="LIMITE" class="Bool"("Blinking"=w1262) -> ()  [unwired: 2 in, 2 out]
              }
              frame True {
                n966 = property on="LIMITE" class="Bool"("Blinking"=w1263) -> ()  [unwired: 2 in, 2 out]
                "LIMITE" <- w1263
              }
            }
            n967 = And(x=w1255, y=w1256) -> (x .and. y?=w1257:bool)
            n968 = case shown="True" w1257 {
              frame False {
              }
              frame True {
                n969 = global write "Global_Telescopio.vi" "AQ Offset Mov"(FALSE ("AQ Offset Mov")) -> ()
              }
            }
            n970 = global read "Global_Telescopio.vi" "Z_SEGURANÇA_GRAUS"() -> (w1254:dbl)
            n971 = global read "Global_Telescopio.vi" "Zenital angle GRAUS"() -> (w1253:dbl)
            n972 = global read "Global_Telescopio.vi" "FinalsFileDownload"() -> (→"Precess Data out-of-date":bool)
            n973 = Greater?(x=w1253, y=w1254) -> (0:→"Security Zone":bool)
          }
          frame #12 {
            w1278 = u16 8 items=["Alarme", "Atencao", "Erro", "Ocupado", "Protecao", "Embreagem", "Tracking", "Var. Track", "Rápido", "Ligeiro", "Médio", "Lento", "Em movimento", ""] ("NomeStatus")
            w1279 = u16 8 items=["Alarme", "Atencao", "Erro", "Ocupado", "Protecao", "Embreagem", "Tracking", "Var. Track", "Rápido", "Ligeiro", "Médio", "Lento", "Em movimento", ""] ("NomeStatus")
            # "ATUALIZAÇÃO DO QUADRO STATUS INFORMATION"
            n974 = call "Bit Status DEC.vi"("NomeStatus"=w1278) -> ("StatBit"=w1276:bool)
            n975 = call "Bit Status AH.vi"("NomeStatus"=w1279) -> ("StatBit"=w1277:bool)
            n976 = global read "Global_Telescopio.vi" "Bit RX Aquis"() -> (w1271:bool)
            n977 = global read "Global_Telescopio.vi" "Bit RX Guider"() -> (w1272:bool)
            n978 = Or(x=w1277, y=w1276) -> (x .or. y?=w1275:bool)
            n979 = case shown="True" w1271 {
              selector: w1271 -> [w1288 w1290]
              frame False {
                n980 = local write "Data Acquisition Activity"(w1288) -> ()
              }
              frame True {
                # "Liga Led RX por 1 ciclo"
                n981 = global write "Global_Telescopio.vi" "Bit RX Aquis"(FALSE) -> ()
                "Data Acquisition Activity" <- w1290
              }
            }
            n982 = case shown="True" w1272 {
              selector: w1272 -> [w1291 w1292]
              frame False {
                n983 = local write "Auto guider Activity"(w1291) -> ()
              }
              frame True {
                # "Liga Led RX por 1 ciclo"
                n984 = global write "Global_Telescopio.vi" "Bit RX Guider"(FALSE) -> ()
                "Auto guider Activity" <- w1292
              }
            }
            n985 = case shown="False" w1275 {
              tunnel: [FALSE w1304] -> w1274
              tunnel: [w1294 w1305] -> w1273
              frame False {
                w1298 = u16 10 items=["Alarme", "Atencao", "Erro", "Ocupado", "Protecao", "Embreagem", "Tracking", "Var. Track", "Rápido", "Ligeiro", "Médio", "Lento", "Em movimento", ""] ("NomeStatus")
                w1297 = u16 10 items=["Alarme", "Atencao", "Erro", "Ocupado", "Protecao", "Embreagem", "Tracking", "Var. Track", "Rápido", "Ligeiro", "Médio", "Lento", "Em movimento", ""] ("NomeStatus")
                w1302 = u16 9 items=["Alarme", "Atencao", "Erro", "Ocupado", "Protecao", "Embreagem", "Tracking", "Var. Track", "Rápido", "Ligeiro", "Médio", "Lento", "Em movimento", ""] ("NomeStatus")
                w1303 = u16 9 items=["Alarme", "Atencao", "Erro", "Ocupado", "Protecao", "Embreagem", "Tracking", "Var. Track", "Rápido", "Ligeiro", "Médio", "Lento", "Em movimento", ""] ("NomeStatus")
                n986 = call "Bit Status AH.vi"("NomeStatus"=w1303) -> ("StatBit"=w1301:bool)
                n987 = call "Bit Status DEC.vi"("NomeStatus"=w1302) -> ("StatBit"=w1300:bool)
                n988 = call "Bit Status AH.vi"("NomeStatus"=w1297) -> ("StatBit"=w1296:bool)
                n989 = call "Bit Status DEC.vi"("NomeStatus"=w1298) -> ("StatBit"=w1295:bool)
                n990 = Compound Arithmetic op=OR(w1301, w1300, w1296, w1295) -> (w1294:bool)
              }
              frame True {
                w1304 = TRUE
                n991 = Not(x=w1304) -> (.not. x?=w1305:bool)
              }
            }
            "Mount Gross Movement" <- w1274
            "Mount Fine Movement" <- w1273
            n992 = case shown="True" "News" {
              selector: "News" -> [_ w1284]
              frame False {
              }
              frame True {
                n993 = flat-sequence {
                  tunnel: w1284 -> [w1285]
                  frame #0 {
                    n994 = call "Monta_Mensagem.vi"("Zerar"=w1285) -> ()  [unwired: 2 in]
                  }
                  frame #1 {
                    n995 = global write "Global_Telescopio.vi" "SYSTEM MESSAGES"("Na janela de SETUP->Configuracao, o endereco do arquivo \"finals2000A.all\" (usado para calculos de  precessao) passou a ser editavel." ("SYSTEM MESSAGES")) -> ()
                  }
                }
              }
            }
            n996 = global read "Global_Telescopio.vi" "SYSTEM MESSAGES"() -> (→"SYSTEM MESSAGES":string)
            n997 = case shown="True" "Clear All Messages" {
              selector: "Clear All Messages" -> [_ w1287]
              frame False {
              }
              frame True {
                n998 = call "Monta_Mensagem.vi"("Zerar"=w1287) -> ()  [unwired: 2 in]
              }
            }
            n999 = local read "alarm Time"() -> (w1266:timestamp)
            n1000 = Get Date/Time In Seconds() -> (seconds since 1Jan1904=w1265:timestamp)
            n1001 = Greater?(x=w1265, y=w1266) -> (0:w1267:bool)
            n1002 = case shown="True" w1267 {
              frame False {
              }
              frame True {
                n1003 = local read "Flag Alarm"() -> (w1280:bool)
                n1004 = case shown="True" w1280 {
                  selector: w1280 -> [_ w1283]
                  frame False {
                  }
                  frame True {
                    n1005 = Not(x=w1283) -> (.not. x?=w1282:bool)
                    n1006 = property on="Mensage Alarme" class="Str"("Visible"=FALSE) -> ()  [unwired: 2 in, 2 out]
                    n1007 = local write "Flag Alarm"(w1282) -> ()
                  }
                }
              }
            }
          }
          frame #13 {
            w1310 = u16 3 items=["Alarme", "Atencao", "Erro", "Ocupado", "Protecao", "Embreagem", "Tracking", "Var. Track", "Rápido", "Ligeiro", "Médio", "Lento", "Em movimento", ""] ("NomeStatus")
            w1311 = u16 3 items=["Alarme", "Atencao", "Erro", "Ocupado", "Protecao", "Embreagem", "Tracking", "Var. Track", "Rápido", "Ligeiro", "Médio", "Lento", "Em movimento", ""] ("NomeStatus")
            # "PROCESSO AQUISIÇÃO"
            n1008 = global read "Global_Telescopio.vi" "Correção Aquis"() -> (w1306:bool)
            n1009 = call "Bit Status AH.vi"("NomeStatus"=w1311) -> ("StatBit"=w1308:bool)
            n1010 = call "Bit Status DEC.vi"("NomeStatus"=w1310) -> ("StatBit"=w1309:bool)
            n1011 = Not Or(1:w1309, 2:w1308) -> (0:w1307:bool)
            n1012 = Compound Arithmetic op=AND(w1306, w1307) -> (w1312:bool)
            n1013 = case shown="True" w1312 {
              frame False {
              }
              frame True {
                # "Reseta Flag do movimento de\n offset do Sist de Aquisição"
                n1014 = global read "Global_Telescopio.vi" "CorrecaoMin"() -> (w1318:dbl)
                n1015 = global read "Global_Telescopio.vi" "aquis_asc"() -> (w1317:dbl)
                n1016 = global read "Global_Telescopio.vi" "aquis_dec"() -> (w1320:dbl)
                n1017 = Absolute Value(x=w1320) -> (abs(x)=w1316:dbl)
                n1018 = global read "Global_Telescopio.vi" "CorrecaoMin"() -> (w1321:dbl)
                n1019 = global write "Global_Telescopio.vi" "Correção Aquis"(FALSE ("Correção Aquis")) -> ()
                n1020 = Absolute Value(x=w1317) -> (abs(x)=w1315:dbl)
                n1021 = Greater?(x=w1316, y=w1321) -> (0:w1322:bool)
                n1022 = Greater?(x=w1315, y=w1318) -> (0:w1319:bool)
                n1023 = case shown="True" w1319 {
                  tunnel: w1317 -> [_ w1323]
                  frame False {
                  }
                  frame True {
                    w1325 = u16 1 items=["ZERO", "AH", "DEC", "TUBO", "CUP"] ("Controlador")
                    # "PROCESSO MOVE TELESCÓPIO"
                    n1024 = call "Conversao Ms to Hora texto.vi"("TRUE=HORA\nFALSE=GRAU"=TRUE ("TRUE=HORA\nFALSE=GRAU"), "PrecDEC"=w1323) -> ("Hora/Graus Texto Decimal"=w1328:string)
                    n1025 = call "Monta Comando.vi"("Set Point"=w1328, "Comando"="MOVER_REL", "Dispositivo"="EIXO" ("Comando"), "Controlador"=w1325) -> ()  [unwired: 3 in, 3 out]
                  }
                }
                n1026 = case shown="True" w1322 {
                  tunnel: w1320 -> [_ w1329]
                  frame False {
                  }
                  frame True {
                    w1331 = u16 2 items=["ZERO", "AH", "DEC", "TUBO", "CUP"] ("Controlador")
                    # "PROCESSO MOVE TELESCÓPIO"
                    n1027 = call "Conversao Ms to Hora texto.vi"("TRUE=HORA\nFALSE=GRAU"=FALSE ("TRUE=HORA\nFALSE=GRAU"), "PrecDEC"=w1329) -> ("Hora/Graus Texto Decimal"=w1334:string)
                    n1028 = call "Monta Comando.vi"("Set Point"=w1334, "Comando"="MOVER_REL", "Dispositivo"="EIXO" ("Comando"), "Controlador"=w1331) -> ()  [unwired: 3 in, 3 out]
                  }
                }
                n1029 = global write "Global_Telescopio.vi" "AQ Offset Mov"(TRUE ("AQ Offset Mov")) -> ()
              }
            }
          }
          frame #14 {
            w1347 = "\r\n"
            # "MUDANÇA 10/8/2010 \nIncluídos:\n- Nome do instrumento\n- RA do telescópio"
            # "OBS: O Arquivo é inicialmente apagado para \nEvitar que fique corrompido!"
            # "Escreve arquivo com Dados para o Uso da Página do PDA"
            n1030 = global read "Global_Telescopio.vi" "Lista Instrumentos"() -> (w1349:string[])
            n1031 = global read "Global_Telescopio.vi" "Sideral Time"() -> (w1339:dbl)
            n1032 = global read "Global_Telescopio.vi" "PosAH"() -> (w1340:dbl)
            n1033 = global read "Global_Telescopio.vi" "Instrum"() -> (w1348:u16)
            n1034 = local read "DOMO_ENC"() -> (w1361:string)
            n1035 = local read "Sideral time"() -> (w1368:string)
            n1036 = local read "CUP_STAT"() -> (w1357:string)
            n1037 = local read "AH_STAT"() -> (w1359:string)
            n1038 = local read "AH_ENC"() -> (w1363:string)
            n1039 = local read "UT"() -> (w1367:string)
            n1040 = Subtract(x=w1339, y=w1340) -> (x-y=w1344:dbl)
            n1041 = Add(x=6.283185307179586, y=w1344) -> (x+y=w1343:dbl)
            n1042 = Less Than 0?(x=w1344) -> (x < 0?=w1341:bool)
            n1043 = call "Retira_tudo_depois_da_virgula.vi"("Entrada"=w1368) -> ("Saída"=w1365:string)
            n1044 = local read "TUBO_STAT"() -> (w1356:string)
            n1045 = Format Date/Time String(time format string (%c)="%H:%M:%S") -> (date/time string=w1351:string)  [unwired: 2 in]
            n1046 = local read "FOCO_ENC"() -> (w1360:string)
            n1047 = local read "DEC_STAT"() -> (w1358:string)
            n1048 = local read "DEC_ENC"() -> (w1362:string)
            n1049 = Select(t=w1343, s=w1341, f=w1344) -> (s? t:f=w1345:dbl)
            n1050 = Index Array(array=w1349, index=w1348) -> (element=w1350:string)
            n1051 = Format Date/Time String(time format string (%c)="%d/%m/%Y") -> (date/time string=w1352:string)  [unwired: 2 in]
            n1052 = call "Retira_tudo_depois_da_virgula.vi"("Entrada"=w1367) -> ("Saída"=w1364:string)
            n1053 = call <vilib>:"Trim Whitespace.vi"("string"=w1365) -> ("trimmed string"=w1355:string)  [unwired: 1 in]
            n1054 = call "rad_hms.vi"("TRUE=HORA\nFALSE=GRAU"=TRUE, "Radiano"=w1345) -> ("Hora/Graus Texto Decimal"=w1338:string)  [unwired: 3 in]
            n1055 = String To Path(string="C:\\TCS\\ARQUIVOS\\DadosTCSPD.txt") -> (path=w1369:path)
            n1056 = Concatenate Strings(w1352, w1347, w1351, w1347, w1364, w1347, w1355, w1347, w1363, w1347, w1362, w1347, w1361, w1347, w1360, w1347, w1359, w1347, w1358, w1347, w1357, w1347, w1356, w1347, w1350, w1347, w1338, w1347) -> (w1371:string)
            n1057 = case shown="True" "Case Constant\n(See Context Help) 2" {
              tunnel: [w1380 w1383] -> w1370
              tunnel: w1369 -> [w1380 w1382]
              frame False {
              }
              frame True {
                n1058 = Delete(path (use dialog)=w1382) -> (deleted path=w1383:path, error out=→"error out":errorcluster)  [unwired: 4 in, 1 out]
              }
            }
            n1059 = call <vilib>:"Open_Create_Replace File.vi"("function (open:0)"=T8."open or create", "file path"=w1370) -> ("error out"=w1375:errorcluster, "refnum"=w1378:refnum<file>)  [unwired: 6 in, 2 out]
            n1060 = Set File Position(refnum=w1378, from (0:start)=enum16{"start", "end", "current"}."start" ("pos mode (0:2)"), error in=w1375) -> (refnum out=w1337:refnum<file>, error out=w1336:errorcluster)  [unwired: 1 in]
            n1061 = Write to Binary File(file (use dialog)=w1337, data=w1371, error in=w1336, 5:FALSE ("prepend array or string size? (T)")) -> (refnum out=w1377:refnum<file>, error out=w1376:errorcluster)  [unwired: 2 in, 1 out]
            n1062 = Close File(refnum=w1377, error in=w1376) -> (error out=w1379:errorcluster)  [unwired: 1 out]
            n1063 = call <vilib>:"Simple Error Handler.vi"("error in (no error)"=w1379) -> ()  [unwired: 4 in, 5 out]
          }
          frame #15 {
            # "Página do PDA"
            # "http://192.168.1.1:1080/pdaWeb/"
            # "TRATAMENTO DO PDA"
            n1064 = stacked-sequence {
              frame #0 {
                # "MUDANÇA  3/9/2010 \nIncluído case abaixo e código de seu estado TRUE para apagar eventuais comandos do PDA enviados antes do TCSPD rodar."
                n1065 = First Call?() -> (First Call?: T/F=w1384:bool)
                n1066 = case shown="True" w1384 {
                  frame False {
                    # "MUDANÇA  4/9/2010 \nSubstituída a VI \"New Read PPC\" pela \"Trata PDA\" a qual evita que o telescópio seja apontado para regiões proibidas (inclinação excessiva)."
                    # "lê e interpreta o arquivo ppc.txt"
